vi "Teste_GirarPlacas.vi"(9 "Angulo Placa 2":dbl, 10 "Angulo Placa 1":dbl, 11 "Inicializar Placas":bool=TRUE) -> (2 "Erro Placa 2":dbl format="%#_13g", 3 "Erro Placa 1":dbl format="%#_13g")   [LabVIEW 2013]
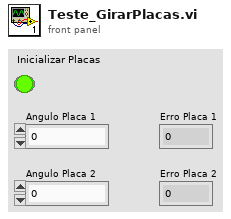
[diagram p1: front panel]
types:
  T1 = cluster{"connection TCP":refnum<k5>, "LogTo File":bool, "Log File refnum":refnum<file>, "no error if error log":bool}
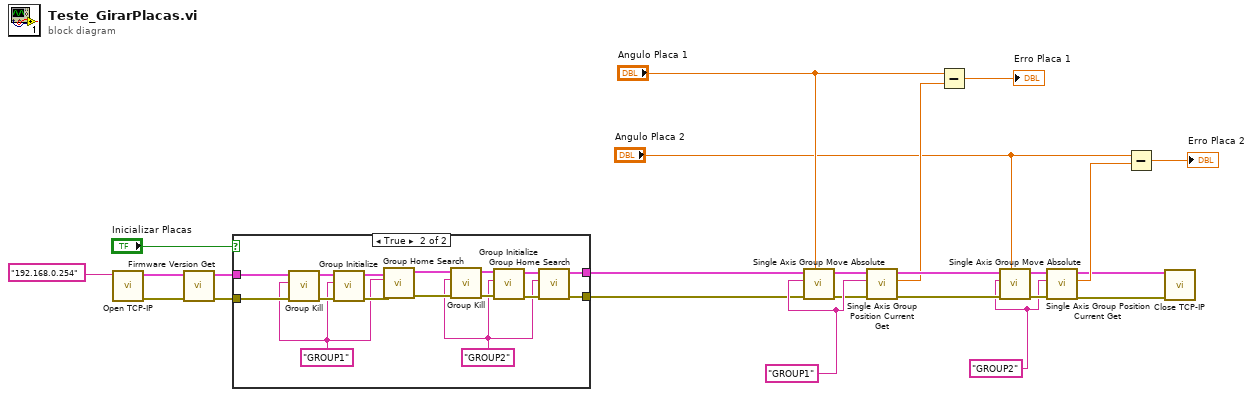
[diagram p0: block diagram]
diagram:
  w17 = "GROUP2" ("Group Name (250 c max)")
  w24 = "GROUP1" ("Group Name (250 c max)")
  n1 = call "Open TCP-IP.vi"("address"="192.168.0.254") -> ("error out"=w13:errorcluster, "Connection ID"=w14:T1)  [unwired: 8 in, 1 out]
  n2 = call "Firmware Version Get.vi"("error in (no error)"=w13, "connection ID in"=w14) -> ("error out"=w10:errorcluster, "connection ID out"=w9:T1)  [unwired: 6 in, 2 out]
  n3 = case shown="True" "Inicializar Placas" {
    tunnel: w9 -> [w26 w31]
    tunnel: w10 -> [w25 w30]
    tunnel: [w26 w29] -> w8
    tunnel: [w25 w28] -> w7
    frame False {
    }
    frame True {
      w27 = "GROUP1" ("Group Name (250 c max)")
      w32 = "GROUP2" ("Group  Name2 (250 c max)")
      n4 = call "Group Kill.vi"("error in (no error)"=w30, "Group Name (250 c max)"=w27, "connection ID in"=w31) -> ("error out"=w42:errorcluster, "connection ID out"=w40:T1)  [unwired: 6 in, 1 out]
      n5 = call "Group Initialize.vi"("error in (no error)"=w42, "Group Name (250 c max)"=w27, "connection ID in"=w40) -> ("error out"=w41:errorcluster, "connection ID out"=w39:T1)  [unwired: 6 in, 1 out]
      n6 = call "Group Home Search.vi"("error in (no error)"=w41, "Group Name (250 c max)"=w27, "connection ID in"=w39) -> ("error out"=w35:errorcluster, "connection ID out"=w38:T1)  [unwired: 6 in, 1 out]
      n7 = call "Group Kill.vi"("error in (no error)"=w35, "Group Name (250 c max)"=w32, "connection ID in"=w38) -> ("error out"=w34:errorcluster, "connection ID out"=w37:T1)  [unwired: 6 in, 1 out]
      n8 = call "Group Initialize.vi"("error in (no error)"=w34, "Group Name (250 c max)"=w32, "connection ID in"=w37) -> ("error out"=w33:errorcluster, "connection ID out"=w36:T1)  [unwired: 6 in, 1 out]
      n9 = call "Group Home Search.vi"("error in (no error)"=w33, "Group Name (250 c max)"=w32, "connection ID in"=w36) -> ("error out"=w28:errorcluster, "connection ID out"=w29:T1)  [unwired: 6 in, 1 out]
    }
  }
  n10 = call "Single Axis Group Move Absolute.vi"("Target Position (units)"="Angulo Placa 1", "error in (no error)"=w7, "Group  Name (250 c max)"=w24, "connection ID in"=w8) -> ("error out"=w22:errorcluster, "connection ID out"=w23:T1)  [unwired: 5 in, 1 out]
  n11 = call "Single Axis Group Position Current Get.vi"("error in (no error)"=w22, "Group  Name (250 c max)"=w24, "connection ID in"=w23) -> ("error out"=w20:errorcluster, "Current Position (units)"=w16:dbl, "connection ID out"=w21:T1)  [unwired: 5 in, 1 out]
  n12 = Subtract(x="Angulo Placa 1", y=w16) -> (x-y=→"Erro Placa 1":dbl)
  n13 = call "Single Axis Group Move Absolute.vi"("Target Position (units)"="Angulo Placa 2", "error in (no error)"=w20, "Group  Name (250 c max)"=w17, "connection ID in"=w21) -> ("error out"=w18:errorcluster, "connection ID out"=w19:T1)  [unwired: 5 in, 1 out]
  n14 = call "Single Axis Group Position Current Get.vi"("error in (no error)"=w18, "Group  Name (250 c max)"=w17, "connection ID in"=w19) -> ("error out"=w1:errorcluster, "Current Position (units)"=w6:dbl, "connection ID out"=w2:T1)  [unwired: 5 in, 1 out]
  n15 = Subtract(x="Angulo Placa 2", y=w6) -> (x-y=→"Erro Placa 2":dbl)
  n16 = call "Close TCP-IP.vi"("error in (no error)"=w1, "connection ID in"=w2) -> ()  [unwired: 9 in, 1 out]
